vi "Dialog_Load positions from PSM.vi"(8 "error in (no error)":errorcluster) -> (0 "error out":errorcluster, 2 "Cancelled or no data?":bool, 3 "Move.to.Pos_Cmd Array":string[](array[string]))   [LabVIEW 2012]
doc: "SciScan 1.2 160622"
uses:
  Dialog_Load positions from PSM_UI Refnums.ctl
  CommonResource VIs/FormatTableStyle_Commands.ctl
  <vilib>/Utility/miscctls.llb/LVRowAndColumnUnsignedTypeDef.ctl
  CommonResource VIs/Timing/Timer Commands.ctl
panel:
  in  "Cancel":bool
  in  "OK":bool
  in  "Notes_Table":string[][](table)
  in  "Big_Table":string[][](table)
  in  "Select/Un-select All":bool=TRUE
  in  "Selection Array":bool[](array[boolean])
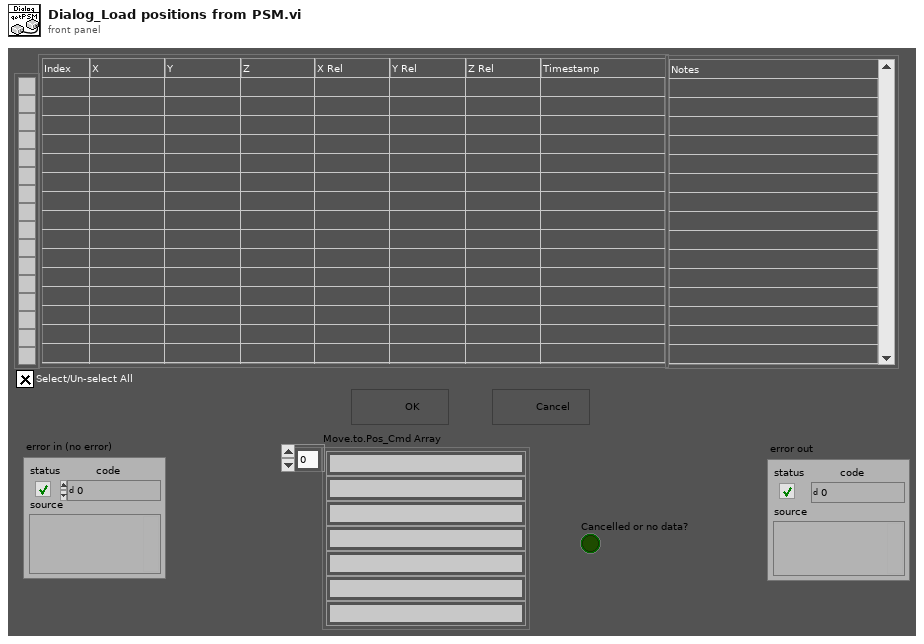
[diagram p1: front panel]
types:
  T1 = typedef "Dialog_Load positions from PSM_UI Refnums.ctl" = cluster{"Big Tbl":refnum<vi>, "Notes Tbl":refnum<vi>, "Sel/Unsel All":refnum<vi>, "Sel. Arr":refnum<vi>}
  T2 = typedef "FormatTableStyle_Commands.ctl" = enum16{"Colour Row", "Uncolour Row", "Bold Row", "Clear table", "UpdateVisibleRows", "Set Row Height", "Enabled Row style", "Disabled Row Style"}
  T3 = typedef "Timer Commands.ctl" = enum16{"Clear All", "Start", "Pause", "Check Time"}
  T4 = typedef "LVRowAndColumnUnsignedTypeDef.ctl" = cluster{"Row":u32, "Column":u32}
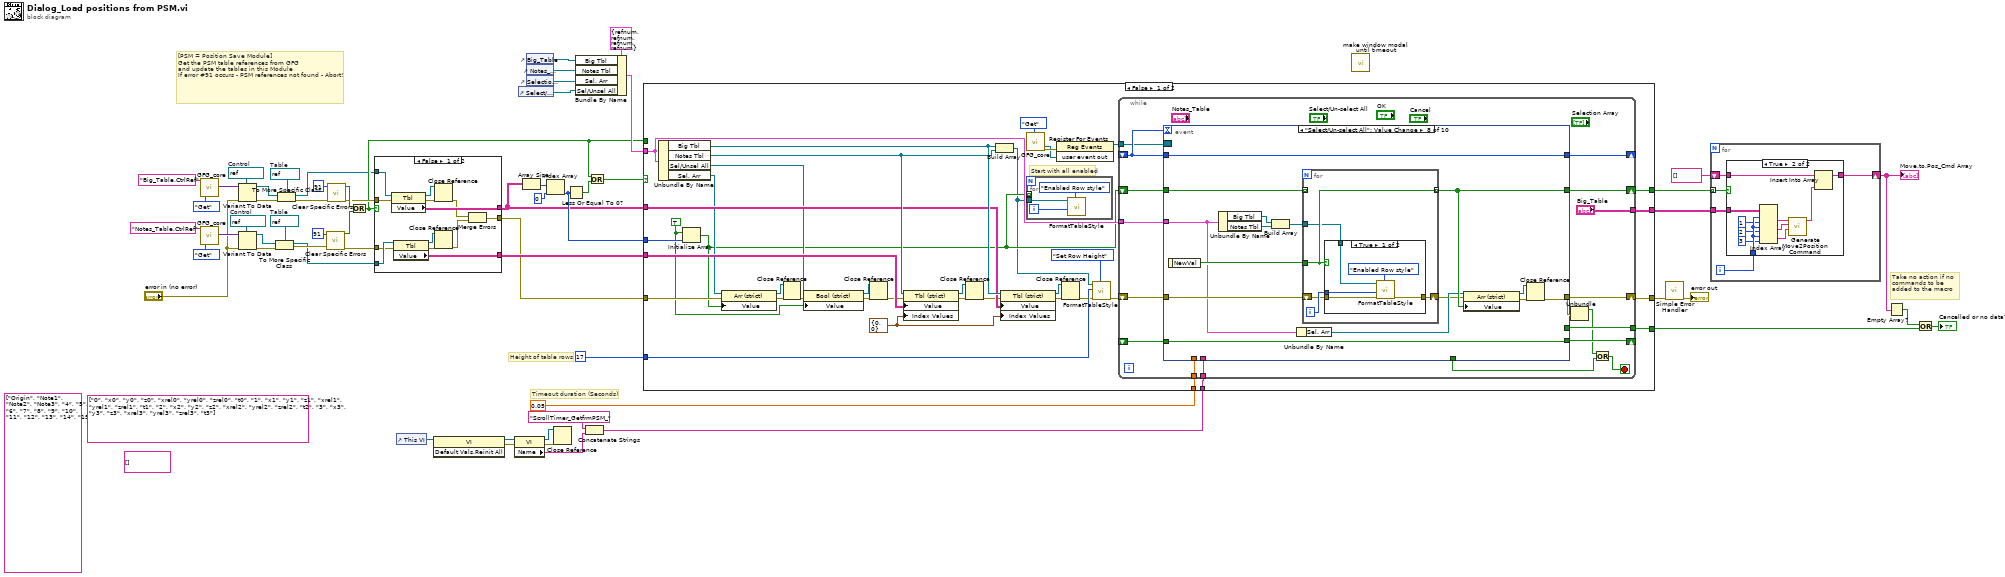
[diagram p0: block diagram]
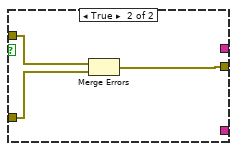
[diagram p2: hidden frame]
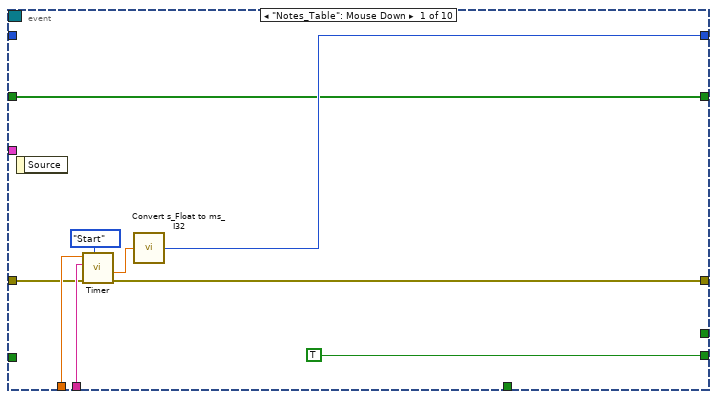
[diagram p4: hidden frame]
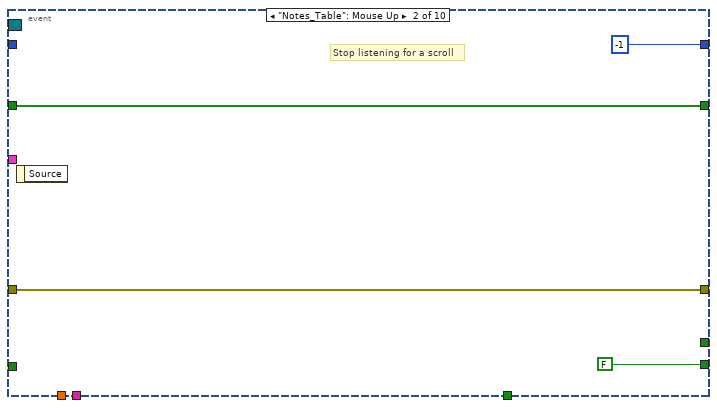
[diagram p5: hidden frame]
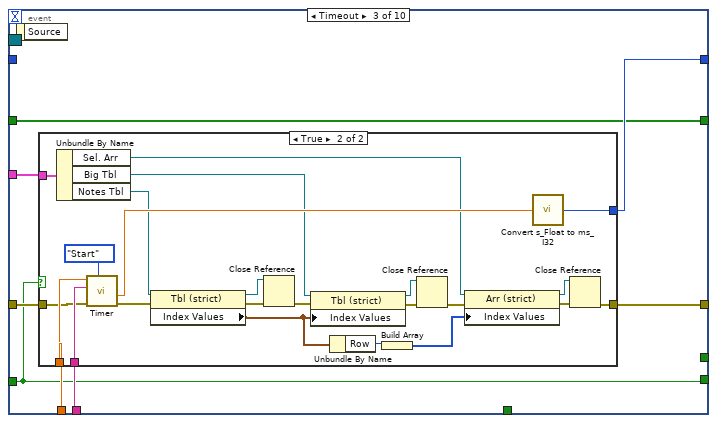
[diagram p6: hidden frame]
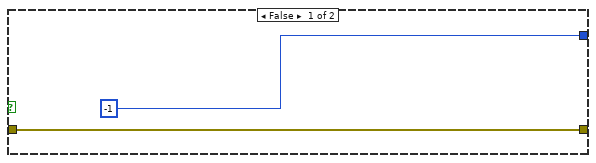
[diagram p7: hidden frame]
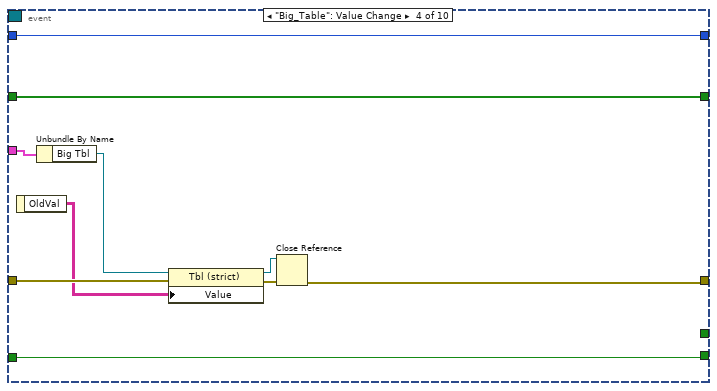
[diagram p8: hidden frame]
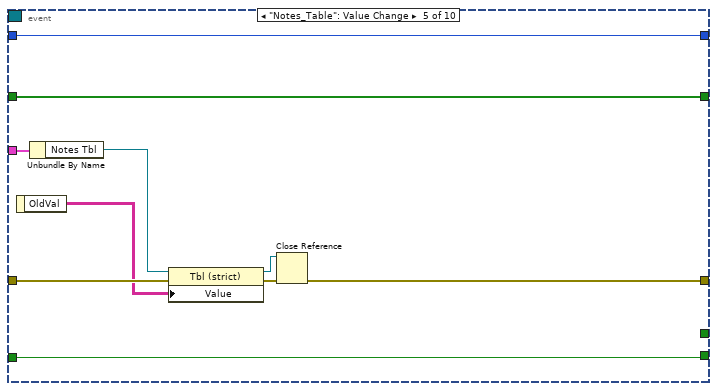
[diagram p9: hidden frame]
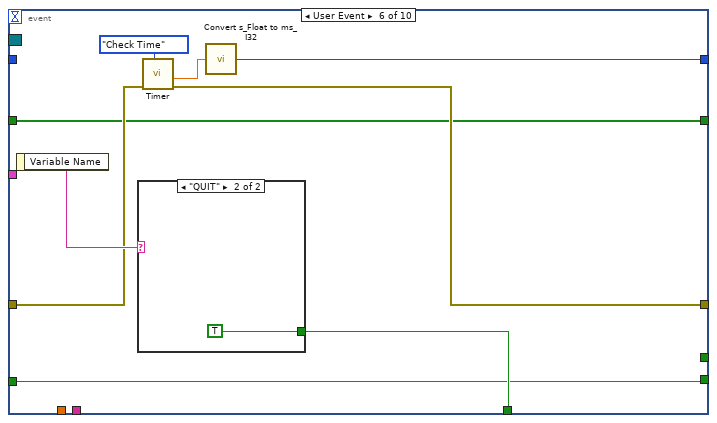
[diagram p10: hidden frame]
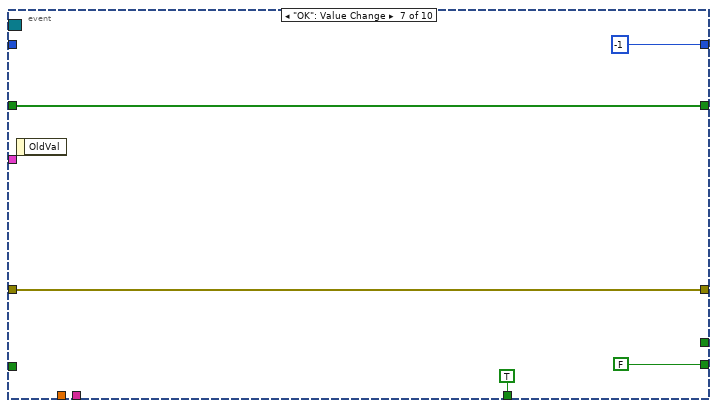
[diagram p12: hidden frame]
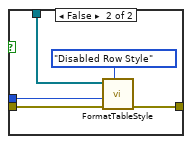
[diagram p13: hidden frame]
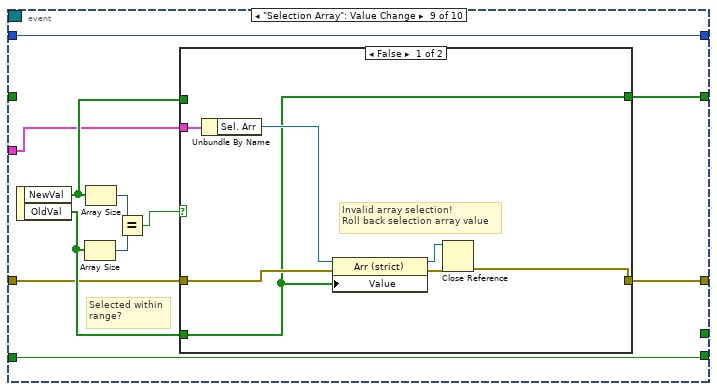
[diagram p14: hidden frame]
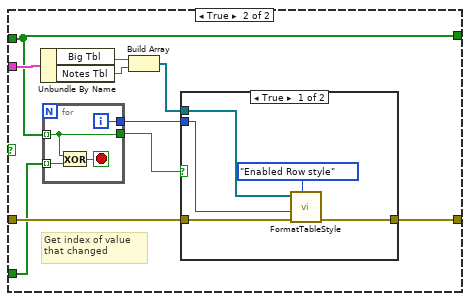
[diagram p15: hidden frame]
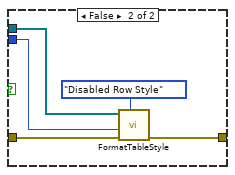
[diagram p16: hidden frame]
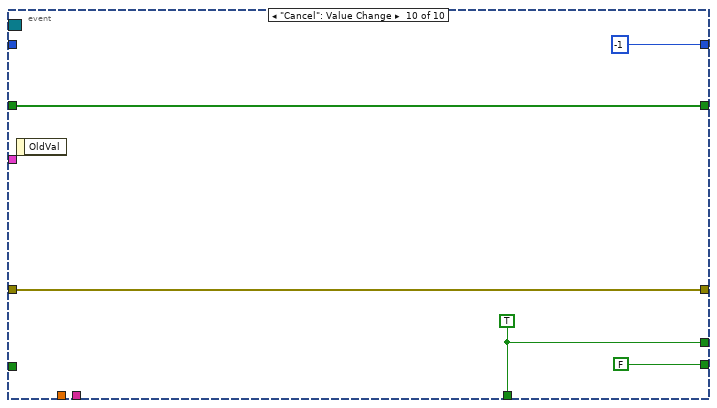
[diagram p17: hidden frame]
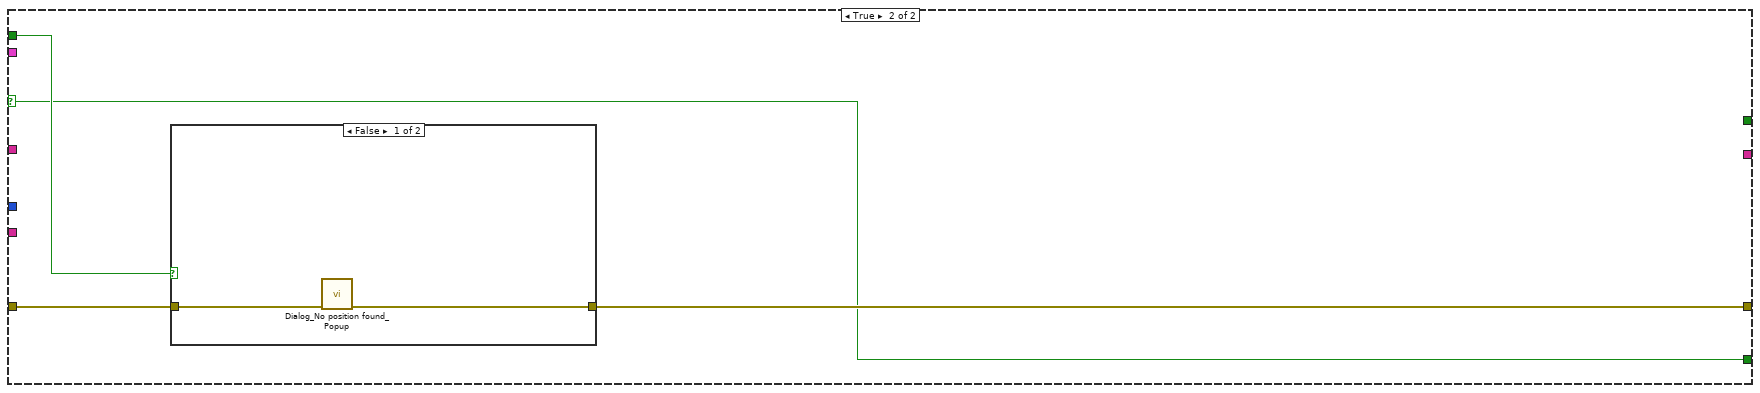
[diagram p18: hidden frame]
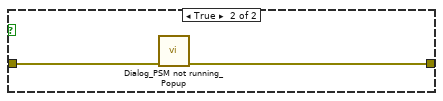
[diagram p19: hidden frame]
diagram:
  w10 = refnum<vi> refnum  # Table
  w14 = refnum<vi> refnum  # Table
  w28 = refnum<vi> refnum  # Control
  w29 = refnum<vi> refnum  # Control
  (unwired) string[][] [] ("Big_Table")
  (unwired) string[][] [["Origin"], ["Note1"], ["Note2"], ["Note3"], ["4"], ["5"], ["6"], ["7"], ["8"], ["9"], ["10"], ["11"], ["12"], ["13"], ["14"], ["15"]] ("Notes_Table")
  (unwired) string[][] [["0", "x0", "y0", "z0", "xrel0", "yrel0", "zrel0", "t0"], ["1", "x1", "y1", "z1", "xrel1", "yrel1", "zrel1", "t1"], ["2", "x2", "y2", "z2", "xrel2", "yrel2", "zrel2", "t2"], ["3", "x3", "y3", "z3", "xrel3", "yrel3", "zrel3", "t3"]] ("Big_Table")
  # "Take no action if no commands to be \nadded to the macro"
  # "[PSM = Position Save Module]\nGet the PSM table references from GFG\nand update the tables in this Module\nIf error #91 occurs - PSM references not found - Abort!"
  # "Timeout duration (Seconds)"
  # "Height of table rows"
  n1 = call "GFG_core.vi"("Variable Name in"="Big_Table.CtrlRef", "Action"=enum16{"Init", "Set", "Get", "Clear"}."Get") -> ("Variant Out"=w31:variant)  [unwired: 11 in, 6 out]
  n2 = call "GFG_core.vi"("Variable Name in"="Notes_Table.CtrlRef", "Action"=enum16{"Init", "Set", "Get", "Clear"}."Get") -> ("Variant Out"=w30:variant)  [unwired: 11 in, 6 out]
  n3 = Variant To Data(error in="error in (no error)", type=w29, Variant=w31) -> (data=w13:refnum<vi>, error out=w11:errorcluster)
  n4 = Variant To Data(error in="error in (no error)", type=w28, Variant=w30) -> (data=w12:refnum<vi>, error out=w9:errorcluster)
  n5 = To More Specific Class(target class=w10, reference=w12, error in=w9) -> (specific class reference=w6:refnum<vi>, error out=w7:errorcluster)
  n6 = To More Specific Class(target class=w14, reference=w13, error in=w11) -> (specific class reference=w8:refnum<vi>, error out=w5:errorcluster)
  n7 = call "Clear Specific Errors.vi"("Error In"=w7, "Error number In"=91) -> ("Error Out"=w22:errorcluster, "Error Cleared?"=w24:bool)  [unwired: 8 in]
  n8 = call "Clear Specific Errors.vi"("Error In"=w5, "Error number In"=91) -> ("Error Out"=w23:errorcluster, "Error Cleared?"=w25:bool)  [unwired: 8 in]
  n9 = Or(x=w25, y=w24) -> (x .or. y?=w15:bool)
  n10 = case shown="False" w15 {
    tunnel: w8 -> [w71 _]
    tunnel: w6 -> [w72 _]
    tunnel: w23 -> [w66 w75]
    tunnel: w22 -> [w65 w74]
    tunnel: [w64 _] -> w21
    tunnel: [w63 _] -> w20
    tunnel: [w60 w73] -> w18
    frame False {
      n11 = property class="Tbl"(reference=w71, error in=w66) -> (reference out=w69:refnum<vi>, error out=w70:errorcluster, "Value"=w64:string[][])
      n12 = property class="Tbl"(reference=w72, error in=w65) -> (reference out=w67:refnum<vi>, error out=w68:errorcluster, "Value"=w63:string[][])
      n13 = Close Reference(reference=w69, error in (no error)=w70) -> (error out=w62:errorcluster)
      n14 = Close Reference(reference=w67, error in (no error)=w68) -> (error out=w61:errorcluster)
      n15 = Merge Errors(w62, w61) -> (w60:errorcluster)
    }
    frame True {
      n16 = Merge Errors(w75, w74) -> (w73:errorcluster)
    }
  }
  n17 = control-ref of="This VI"() -> (w44:refnum<vi>)
  n18 = invoke class="VI" method="Default Vals.Reinit All"(reference=w44) -> (reference out=w42:refnum<vi>, error out=w43:errorcluster)  [unwired: 2 in, 1 out]
  n19 = property class="VI"(reference=w42, error in=w43) -> (reference out=w48:refnum<vi>, error out=w49:errorcluster, "Name"=w47:string)
  n20 = control-ref of="Select/Un-select All"() -> (w55:refnum<vi>)
  n21 = Array Size(array=w21) -> (size(s)=w54:i32[])
  n22 = control-ref of="Big_Table"() -> (w58:refnum<vi>)
  n23 = control-ref of="Notes_Table"() -> (w57:refnum<vi>)
  n24 = control-ref of="Selection Array"() -> (w56:refnum<vi>)
  n25 = Index Array(array=w54, index=0) -> (element=w39:i32)
  n26 = Close Reference(reference=w48, error in (no error)=w49) -> ()  [unwired: 1 out]
  n27 = Less Or Equal To 0?(x=w39) -> (x <= 0?=w17:bool)
  n28 = Bundle By Name(cluster=T1 {"Big Tbl"=refnum, "Notes Tbl"=refnum, "Sel/Unsel All"=refnum, "Sel. Arr"=refnum} ("Dialog_Load positions from PSM_UI Refnums"), "Big Tbl"=w58, "Notes Tbl"=w57, "Sel. Arr"=w56, "Sel/Unsel All"=w55) -> (w52:T1)
  n29 = Concatenate Strings("ScrollTimer_GetfrmPSM_", w47) -> (w46:string)
  n30 = Or(x=w15, y=w17) -> (x .or. y?=w16:bool)
  n31 = case shown="False" w16 {
    selector: w16 -> [_ w292]
    tunnel: w52 -> [w93 _]
    tunnel: w18 -> [w88 w295]
    tunnel: u32 17 ("Active Cell:Cell Size:Height 2") -> [w113 _]
    tunnel: w20 -> [w110 _]
    tunnel: w21 -> [w108 _]
    tunnel: [w92 w293] -> w41
    tunnel: w46 -> [w99 _]
    tunnel: 0.05 ("Set Time IN (s)") -> [w98 _]
    tunnel: [w91 w292] -> w2
    tunnel: w39 -> [w90 _]
    tunnel: [w79 _] -> w37
    tunnel: [w78 _] -> w38
    tunnel: w15 -> [_ w294]
    frame False {
      w83 = TRUE
      w101 = T4 {"Row"=0, "Column"=0} ("Index Values")
      # "Start with all enabled"
      n32 = Unbundle By Name(w93) -> ("Big Tbl"=w109:refnum<vi>, "Notes Tbl"=w111:refnum<vi>, "Sel/Unsel All"=w84:refnum<vi>, "Sel. Arr"=w89:refnum<vi>)
      n33 = Initialize Array(w83, w90) -> (w77:bool[])
      n34 = property class="Arr (strict)"(reference=w89, error in=w88, "Value"=w77) -> (reference out=w86:refnum<vi>, error out=w87:errorcluster)
      n35 = Close Reference(reference=w86, error in (no error)=w87) -> (error out=w85:errorcluster)
      n36 = property class="Bool (strict)"(reference=w84, error in=w85, "Value"=w83) -> (reference out=w81:refnum<vi>, error out=w82:errorcluster)
      n37 = Close Reference(reference=w81, error in (no error)=w82) -> (error out=w80:errorcluster)
      n38 = property class="Tbl (strict)"(reference=w111, error in=w80, "Value"=w110, "Index Values"=w101) -> (reference out=w106:refnum<vi>, error out=w107:errorcluster)
      n39 = Close Reference(reference=w106, error in (no error)=w107) -> (error out=w105:errorcluster)
      n40 = Build Array(w109, w111) -> (w76:refnum<vi>[])
      n41 = property class="Tbl (strict)"(reference=w109, error in=w105, "Value"=w108, "Index Values"=w101) -> (reference out=w103:refnum<vi>, error out=w104:errorcluster)
      n42 = call "GFG_core.vi"("Action"=enum16{"Init", "Set", "Get", "Clear"}."Get") -> ("user event out"=w95:refnum<user-event>, "error out"=w96:errorcluster)  [unwired: 12 in, 5 out]
      n43 = for {
        tunnel: w77 -> [_] mode=indexing
        tunnel: w76 -> [w114]
        i -> [w115]
        n44 = call "FormatTableStyle.vi"("Format Command"=FormatTableStyle_Commands."Enabled Row style", "Row Index"=w115, "Table reference Array"=w114) -> ()  [unwired: 8 in, 1 out]
      }
      n45 = register-events(error in=w96, w95) -> (reference out=w94:refnum<event-registration>)  [unwired: 1 in, 1 out]
      n46 = Close Reference(reference=w103, error in (no error)=w104) -> (error out=w102:errorcluster)
      n47 = call "FormatTableStyle.vi"("Format Command"=FormatTableStyle_Commands."Set Row Height", "Error In"=w102, "Parameter (Optional)"=w113, "Table reference Array"=w76) -> ("Error Out"=w100:errorcluster)  [unwired: 7 in]
      n48 = while {
        tunnel: w99 -> [w132]
        tunnel: w98 -> [w131]
        shift-right: [w130] -> _
        shift-left: _ -> [w129]
        shift-right: [w128] -> _
        shift-left: _ -> [w127]
        tunnel: w94 -> [w126]
        tunnel: w93 -> [w125]
        tunnel: [w124] -> w91
        shift-right: [w123] -> w92
        shift-left: w100 -> [w133]
        tunnel: ["Big_Table"] -> w78
        shift-right: [w118] -> w79
        shift-left: w77 -> [w117]
        stop <- w120 stop-if-true
        n49 = event shown="[7] \"Select/Un-select All\": Value Change" {
          selector: w126 -> [_ _ _ _ _ _ _ _ _ _]
          dyn-events: _ -> [_ _ _ _ _ _ _ _ _ _]
          timeout: w127 -> [_ _ _ _ _ _ _ _ _ _]
          tunnel: w133 -> [w136 w144 w153 w186 w196 w204 w211 w221 w248 w290]
          tunnel: w132 -> [w140 _ w151 _ _ _ _ _ _ _]
          tunnel: w131 -> [w139 _ w152 _ _ _ _ _ _ _]
          tunnel: [TRUE FALSE w150 w181 w191 w202 FALSE w225 w255 FALSE] -> w130
          tunnel: w129 -> [_ _ w150 w181 w191 w202 _ w225 w255 _]
          tunnel: [w137 -1 ("milliseconds OUT (I32)") w149 w180 w190 w203 -1 ("milliseconds OUT (I32)") w224 w254 -1 ("milliseconds OUT (I32)")] -> w128
          tunnel: w127 -> [_ _ _ w180 w190 _ _ w224 w254 _]
          tunnel: [_ _ _ _ _ w205 TRUE _ _ w288] -> w121
          tunnel: w125 -> [_ _ w154 w188 w198 _ _ w218 w247 _]
          tunnel: [w135 w144 w148 w182 w192 w201 w211 w226 w245 w290] -> w123
          tunnel: [_ _ _ _ _ _ _ _ _ w288] -> w124
          tunnel: [w134 w143 w147 w189 w199 w200 w210 w223 w246 w287] -> w118
          tunnel: w117 -> [w134 w143 w147 w189 w199 w200 w210 w219 _ w287]
          event "Notes_Table": Mouse Down {
            n50 = event-data() -> ()  [unwired: 1 in, 1 out]
            n51 = call "Timer.vi"("Timer Command"=Timer_Commands."Start", "Error In"=w136, "VI name (Optional)"=w140, "Set Time IN (s)"=w139) -> ("Error Out"=w135:errorcluster, "Remaining Time (s)"=w141:dbl)  [unwired: 2 in, 4 out]
            n52 = call "Convert s_Float to ms_I32.vi"("Seconds IN (Float)"=w141) -> ("milliseconds OUT (I32)"=w137:i32)
          }
          event "Notes_Table": Mouse Up {
            # "Stop listening for a scroll"
            n53 = event-data() -> ()  [unwired: 1 in, 1 out]
          }
          event Timeout {
            n54 = event-data() -> ()  [unwired: 1 in, 1 out]
            n55 = case shown="True" w150 {
              tunnel: w151 -> [_ w179]
              tunnel: w152 -> [_ w178]
              tunnel: [-1 ("milliseconds OUT (I32)") w175] -> w149
              tunnel: w153 -> [w155 w169]
              tunnel: w154 -> [_ w167]
              tunnel: [w155 w157] -> w148
              frame False {
              }
              frame True {
                n56 = Unbundle By Name(w167) -> ("Sel. Arr"=w163:refnum<vi>, "Big Tbl"=w162:refnum<vi>, "Notes Tbl"=w170:refnum<vi>)
                n57 = call "Timer.vi"("Timer Command"=Timer_Commands."Start", "Error In"=w169, "VI name (Optional)"=w179, "Set Time IN (s)"=w178) -> ("Error Out"=w168:errorcluster, "Remaining Time (s)"=w176:dbl)  [unwired: 2 in, 4 out]
                n58 = property class="Tbl (strict)"(reference=w170, error in=w168) -> (reference out=w172:refnum<vi>, error out=w171:errorcluster, "Index Values"=w160:T4)
                n59 = Close Reference(reference=w172, error in (no error)=w171) -> (error out=w164:errorcluster)
                n60 = property class="Tbl (strict)"(reference=w162, error in=w164, "Index Values"=w160) -> (reference out=w165:refnum<vi>, error out=w166:errorcluster)
                n61 = Unbundle By Name(w160) -> ("Row"=w159:u32)
                n62 = Build Array(w159) -> (w158:u32[])
                n63 = Close Reference(reference=w165, error in (no error)=w166) -> (error out=w161:errorcluster)
                n64 = property class="Arr (strict)"(reference=w163, error in=w161, "Index Values"=w158) -> (reference out=w174:refnum<vi>, error out=w173:errorcluster)
                n65 = call "Convert s_Float to ms_I32.vi"("Seconds IN (Float)"=w176) -> ("milliseconds OUT (I32)"=w175:i32)
                n66 = Close Reference(reference=w174, error in (no error)=w173) -> (error out=w157:errorcluster)
              }
            }
          }
          event "Big_Table": Value Change {
            n67 = event-data() -> ("OldVal"=w185:string[][])  [unwired: 1 in]
            n68 = Unbundle By Name(w188) -> ("Big Tbl"=w187:refnum<vi>)
            n69 = property class="Tbl (strict)"(reference=w187, error in=w186, "Value"=w185) -> (reference out=w183:refnum<vi>, error out=w184:errorcluster)
            n70 = Close Reference(reference=w183, error in (no error)=w184) -> (error out=w182:errorcluster)
          }
          event "Notes_Table": Value Change {
            n71 = event-data() -> ("OldVal"=w195:string[][])  [unwired: 1 in]
            n72 = Unbundle By Name(w198) -> ("Notes Tbl"=w197:refnum<vi>)
            n73 = property class="Tbl (strict)"(reference=w197, error in=w196, "Value"=w195) -> (reference out=w193:refnum<vi>, error out=w194:errorcluster)
            n74 = Close Reference(reference=w193, error in (no error)=w194) -> (error out=w192:errorcluster)
          }
          event User Event {
            n75 = event-data() -> ("Variable Name"=w206:string)  [unwired: 1 in]
            n76 = case shown="\"QUIT\"" w206 {
              tunnel: [_ TRUE] -> w205
              frame Default {
              }
              frame "QUIT" {
              }
            }
            n77 = call "Timer.vi"("Timer Command"=Timer_Commands."Check Time", "Error In"=w204) -> ("Error Out"=w201:errorcluster, "Remaining Time (s)"=w207:dbl)  [unwired: 4 in, 4 out]
            n78 = call "Convert s_Float to ms_I32.vi"("Seconds IN (Float)"=w207) -> ("milliseconds OUT (I32)"=w203:i32)
          }
          event "OK": Value Change {
            n79 = event-data() -> ()  [unwired: 1 in, 1 out]
          }
          event "Select/Un-select All": Value Change {
            n80 = event-data() -> ("NewVal"=w229:bool)  [unwired: 1 in]
            n81 = Unbundle By Name(w218) -> ("Big Tbl"=w217:refnum<vi>, "Notes Tbl"=w216:refnum<vi>)
            n82 = Build Array(w217, w216) -> (w215:refnum<vi>[])
            n83 = Unbundle By Name(w218) -> ("Sel. Arr"=w222:refnum<vi>)
            n84 = for {
              tunnel: w229 -> [w234]
              tunnel: [w234] -> w223 mode=indexing
              shift-right: [w231] -> w220
              shift-left: w221 -> [w232]
              tunnel: w219 -> [_] mode=indexing
              tunnel: w215 -> [w230]
              i -> [w233]
              n85 = case shown="True" w234 {
                tunnel: w233 -> [w238 w242]
                tunnel: w232 -> [w237 w243]
                tunnel: [w236 w241] -> w231
                tunnel: w230 -> [w235 w240]
                frame True {
                  n86 = call "FormatTableStyle.vi"("Format Command"=FormatTableStyle_Commands."Enabled Row style", "Error In"=w237, "Row Index"=w238, "Table reference Array"=w235) -> ("Error Out"=w236:errorcluster)  [unwired: 7 in]
                }
                frame False {
                  n87 = call "FormatTableStyle.vi"("Format Command"=FormatTableStyle_Commands."Disabled Row Style", "Error In"=w243, "Row Index"=w242, "Table reference Array"=w240) -> ("Error Out"=w241:errorcluster)  [unwired: 7 in]
                }
              }
            }
            n88 = property class="Arr (strict)"(reference=w222, error in=w220, "Value"=w223) -> (reference out=w227:refnum<vi>, error out=w228:errorcluster)
            n89 = Close Reference(reference=w227, error in (no error)=w228) -> (error out=w226:errorcluster)
          }
          event "Selection Array": Value Change {
            # "Selected within\nrange?"
            n90 = event-data() -> ("NewVal"=w249:bool[], "OldVal"=w250:bool[])  [unwired: 1 in]
            n91 = Array Size(array=w250) -> (size(s)=w252:i32)
            n92 = Array Size(array=w249) -> (size(s)=w253:i32)
            n93 = Equal?(x=w253, y=w252) -> (x = y?=w251:bool)
            n94 = case shown="False" w251 {
              tunnel: w247 -> [w262 w272]
              tunnel: w248 -> [w257 w271]
              tunnel: [w258 w270] -> w245
              tunnel: w249 -> [_ w264]
              tunnel: w250 -> [w256 w269]
              tunnel: [w256 w264] -> w246
              frame False {
                # "Invalid array selection!\nRoll back selection array value"
                n95 = Unbundle By Name(w262) -> ("Sel. Arr"=w261:refnum<vi>)
                n96 = property class="Arr (strict)"(reference=w261, error in=w257, "Value"=w256) -> (reference out=w259:refnum<vi>, error out=w260:errorcluster)
                n97 = Close Reference(reference=w259, error in (no error)=w260) -> (error out=w258:errorcluster)
              }
              frame True {
                # "Get index of value that changed"
                n98 = Unbundle By Name(w272) -> ("Big Tbl"=w266:refnum<vi>, "Notes Tbl"=w265:refnum<vi>)
                n99 = for {
                  tunnel: w264 -> [w283] mode=indexing
                  tunnel: w269 -> [w286] mode=indexing
                  tunnel: [w284] -> w268
                  tunnel: [w283] -> w267
                  i -> [w284]
                  stop <- w285 stop-if-true
                  n100 = Exclusive Or(1:w286, 2:w283) -> (0:w285:bool)
                }
                n101 = Build Array(w266, w265) -> (w263:refnum<vi>[])
                n102 = case shown="True" w267 {
                  tunnel: w271 -> [w276 w281]
                  tunnel: w268 -> [w274 w279]
                  tunnel: w263 -> [w275 w280]
                  tunnel: [w273 w278] -> w270
                  frame True {
                    n103 = call "FormatTableStyle.vi"("Format Command"=FormatTableStyle_Commands."Enabled Row style", "Error In"=w276, "Row Index"=w274, "Table reference Array"=w275) -> ("Error Out"=w273:errorcluster)  [unwired: 7 in]
                  }
                  frame False {
                    n104 = call "FormatTableStyle.vi"("Format Command"=FormatTableStyle_Commands."Disabled Row Style", "Error In"=w281, "Row Index"=w279, "Table reference Array"=w280) -> ("Error Out"=w278:errorcluster)  [unwired: 7 in]
                  }
                }
              }
            }
          }
          event "Cancel": Value Change {
            w288 = TRUE
            n105 = event-data() -> ()  [unwired: 1 in, 1 out]
          }
        }
        n106 = Unbundle(w123) -> ("status"=w122:bool)  [unwired: 2 out]
        n107 = Or(x=w122, y=w121) -> (x .or. y?=w120:bool)
      }
    }
    frame True {
      n108 = case shown="False" w294 {
        tunnel: w295 -> [w297 w299]
        tunnel: [w296 w298] -> w293
        frame False {
          n109 = call "Dialog_No position found_Popup.vi"("error in (no error)"=w297) -> ("error out"=w296:errorcluster)  [unwired: 10 in]
        }
        frame True {
          n110 = call "Dialog_PSM not running_Popup.vi"("error in (no error)"=w299) -> ("error out"=w298:errorcluster)  [unwired: 10 in]
        }
      }
    }
  }
  n111 = call "make window modal until timeout.vi"() -> ()  [unwired: 12 in]
  n112 = call <vilib>:"Simple Error Handler.vi"("error in (no error)"=w41) -> ("error out"=→"error out":errorcluster)  [unwired: 4 in, 4 out]
  n113 = for {
    tunnel: w38 -> [w304]
    tunnel: w37 -> [w302] mode=indexing
    shift-right: [w300] -> w4
    shift-left: string[] [] -> [w301]
    i -> [w303]
    n114 = case shown="True" w302 {
      tunnel: w304 -> [_ w316]
      tunnel: w303 -> [_ w315]
      tunnel: w301 -> [w305 w307]
      tunnel: [w305 w306] -> w300
      frame False {
      }
      frame True {
        n115 = Index Array(array=w316, index (row) #1=w315, index (col) #1=1 ("disabled index (col)"), index (row) #2=w315, index (col) #2=2 ("disabled index (col)"), index (row) #3=w315, index (col) #3=3 ("disabled index (col)")) -> (element #1=w311:string, element #2=w310:string, element #3=w309:string)
        n116 = call "Generate Move2Position Command.vi"("Pos.Z(um)"=w309, "Pos.Y(um)"=w310, "Pos.X(um)"=w311) -> ("Move2Position Command OUT"=w308:string)  [unwired: 7 in, 1 out]
        n117 = Insert Into Array(array=w307, new element=w308) -> (w306:string[])  [unwired: 1 in]
      }
    }
  }
  "Move.to.Pos_Cmd Array" <- w4
  n118 = Empty Array?(array=w4) -> (empty?=w3:bool)
  n119 = Or(x=w3, y=w2) -> (x .or. y?=→"Cancelled or no data?":bool)
